vi "Update State Name in Channel Value Table.vi"(8 "error in (no error)":errorcluster, 9 "New State Name":string, 10 "State":string, 11 "Channel Ref in":T1 format="%.0x") -> (0 "error out":errorcluster, 3 "Channel Ref out":T1=18446744073709551615 format="%.0x")   [LabVIEW 2017, in "Switch Scripting.lvlib"]
uses:
  Switch Scripting.lvlib
  <vilib>/NI Veristand/Custom Device API/Custom Device Item Ref.ctl
  <vilib>/NI VeriStand/Custom Device API/Custom Device API.lvlib
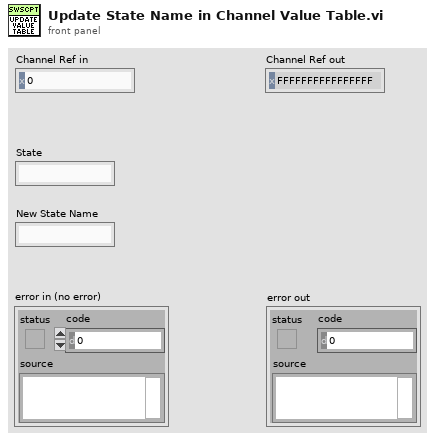
[diagram p1: front panel]
types:
  T1 = typedef "Custom Device API.lvlib/Custom Device Item Ref.ctl" = u64
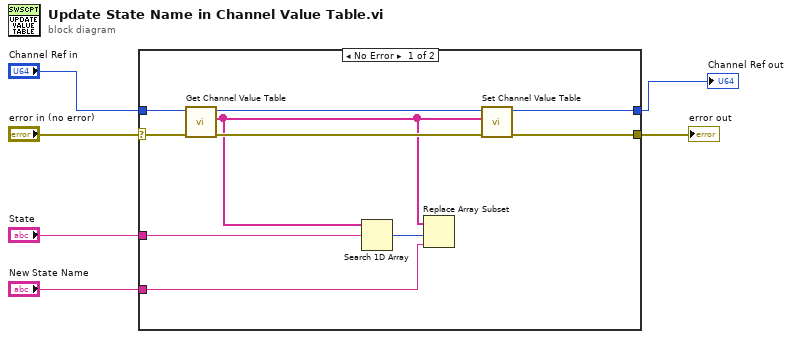
[diagram p0: block diagram]
diagram:
  n1 = case shown="No Error" "error in (no error)" {
    selector: "error in (no error)" -> [w15 w18]
    tunnel: [w10 w18] -> w3
    tunnel: "Channel Ref in" -> [w12 w17]
    tunnel: [w11 w17] -> w4
    tunnel: "State" -> [w16 _]
    tunnel: "New State Name" -> [w7 _]
    frame No Error {
      n2 = call "Get Channel Value Table.vi"("error in (no error)"=w15, "Channel Ref in"=w12) -> ("error out"=w14:errorcluster, "States"=w8:string[], "Channel Ref out"=w13:T1)  [unwired: 6 in, 1 out]
      n3 = Search 1D Array(1D array=w8, element=w16) -> (index of element=w9:i32)  [unwired: 1 in]
      n4 = Replace Array Subset(array=w8, new element=w7, index=w9) -> ()  [unwired: 1 out]
      n5 = call "Set Channel Value Table.vi"("error in (no error)"=w14, "States"=w8, "Channel Ref in"=w13) -> ("error out"=w10:errorcluster, "Channel Ref out"=w11:T1)  [unwired: 7 in]
    }
    frame Error {
    }
  }
  "Channel Ref out" <- w4
  "error out" <- w3
